vi "path2str.vi"(0 "options file":path, 1 "keyringfile":path, 2 "Sec keyringfile":path, 3 "Trust DB":path, 4 "targetfile":path, 5 "sourcefile":path) -> (10 "tf NaPath":bool, 12 "sf NaPath":bool, 14 "options path":string, 15 "keyringfile path":string, 16 "Trust DB path":string, 17 "opt/keyr/seckeyr/trusdb":string, 18 "targetfile path":string, 19 "sourcefile path":string)   [LabVIEW 2012, in "HGF_GPG.lvlib" / "HGF_GPG.lvclass"]
uses:
  HGF_GPG.lvclass
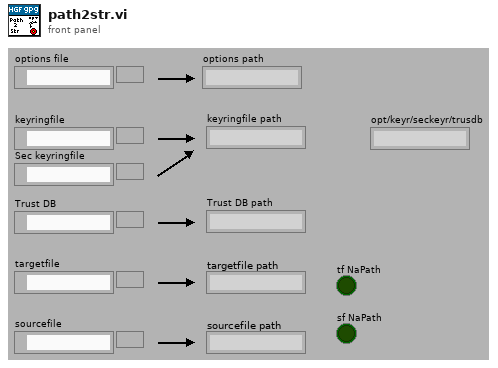
[diagram p1: front panel]
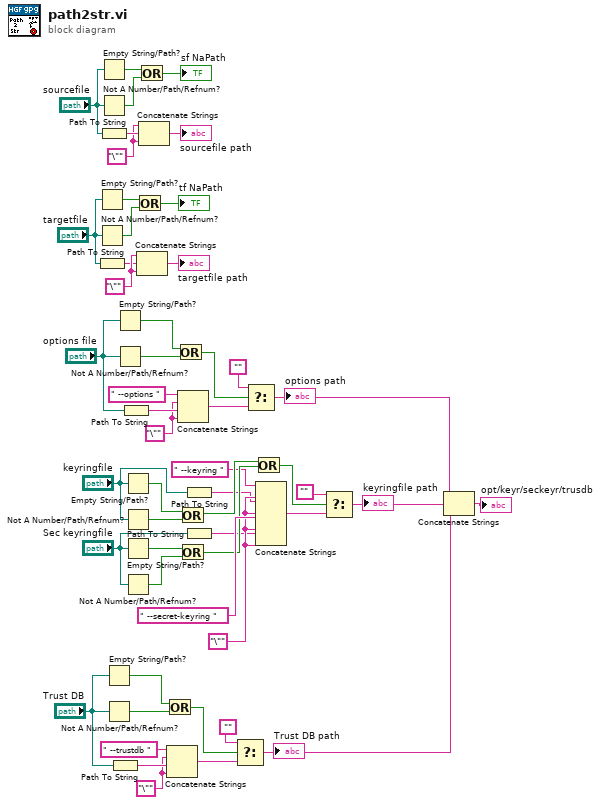
[diagram p0: block diagram]
diagram:
  w7 = "\""
  w20 = "\""
  w28 = "\""
  w49 = "\""
  w48 = "\""
  n1 = Empty String/Path?(string/path="targetfile") -> (empty?=w37:bool)
  n2 = Not A Number/Path/Refnum?(number/path/refnum="targetfile") -> (NaN/Path/Refnum?=w38:bool)
  n3 = Path To String(path="targetfile") -> (string=w47:string)
  n4 = Empty String/Path?(string/path="sourcefile") -> (empty?=w26:bool)
  n5 = Not A Number/Path/Refnum?(number/path/refnum="sourcefile") -> (NaN/Path/Refnum?=w25:bool)
  n6 = Path To String(path="sourcefile") -> (string=w21:string)
  n7 = Empty String/Path?(string/path="Trust DB") -> (empty?=w11:bool)
  n8 = Not A Number/Path/Refnum?(number/path/refnum="Trust DB") -> (NaN/Path/Refnum?=w10:bool)
  n9 = Path To String(path="Trust DB") -> (string=w14:string)
  n10 = Empty String/Path?(string/path="options file") -> (empty?=w32:bool)
  n11 = Not A Number/Path/Refnum?(number/path/refnum="options file") -> (NaN/Path/Refnum?=w33:bool)
  n12 = Path To String(path="options file") -> (string=w29:string)
  n13 = Empty String/Path?(string/path="keyringfile") -> (empty?=w36:bool)
  n14 = Not A Number/Path/Refnum?(number/path/refnum="keyringfile") -> (NaN/Path/Refnum?=w35:bool)
  n15 = Empty String/Path?(string/path="Sec keyringfile") -> (empty?=w17:bool)
  n16 = Not A Number/Path/Refnum?(number/path/refnum="Sec keyringfile") -> (NaN/Path/Refnum?=w16:bool)
  n17 = Or(x=w37, y=w38) -> (x .or. y?=→"tf NaPath":bool)
  n18 = Or(x=w26, y=w25) -> (x .or. y?=→"sf NaPath":bool)
  n19 = Concatenate Strings(w48, w47, w48) -> (→"targetfile path":string)
  n20 = Concatenate Strings(w20, w21, w20) -> (→"sourcefile path":string)
  n21 = Or(x=w11, y=w10) -> (x .or. y?=w9:bool)
  n22 = Concatenate Strings(" --trustdb " ("string"), w7, w14, w7) -> (w12:string)
  n23 = Or(x=w32, y=w33) -> (x .or. y?=w34:bool)
  n24 = Concatenate Strings(" --options " ("string"), w28, w29, w28) -> (w31:string)
  n25 = Or(x=w36, y=w35) -> (x .or. y?=w51:bool)
  n26 = Or(x=w17, y=w16) -> (x .or. y?=w50:bool)
  n27 = Path To String(path="keyringfile") -> (string=w46:string)
  n28 = Path To String(path="Sec keyringfile") -> (string=w19:string)
  n29 = Select(t="" ("f"), s=w9, f=w12) -> (s? t:f=w2:string)
  "Trust DB path" <- w2
  n30 = Select(t="" ("f"), s=w34, f=w31) -> (s? t:f=w4:string)
  "options path" <- w4
  n31 = Or(x=w51, y=w50) -> (x .or. y?=w15:bool)
  n32 = Concatenate Strings(" --keyring " ("string"), w49, w46, w49, " --secret-keyring " ("string"), w49, w19, w49) -> (w44:string)
  n33 = Select(t="" ("f"), s=w15, f=w44) -> (s? t:f=w3:string)
  "keyringfile path" <- w3
  n34 = Concatenate Strings(w4, w3, w2) -> (→"opt/keyr/seckeyr/trusdb":string)
